vi "WPI_AnalogChannelGetOffset.vi"(8 "error in (no error)":errorcluster, 11 "AIDeviceRef":T1={"DevStatus"={"status"=FALSE, "code"=0, "source"=""}, "Analog Channel"=enum."Invalid"}) -> (0 "error out":errorcluster, 2 "Offset":dbl, 3 "AIDeviceRef":T1={"DevStatus"={"status"=FALSE, "code"=0, "source"=""}, "Analog Channel"=enum."Invalid"})   [LabVIEW 2017]
doc: "Returns the factory offset value that the A/D converter uses to scale the signal.\n\nThis software is licensed. Open the labview\\readme\\WPI Robotics Library Open Source License.txt file for more information."
uses:
  <vilib>/Rock Robotics/WPI/AnalogChannel/WPI_AnalogChannelDevRef.ctl
  <vilib>/Rock Robotics/SystemInterfaces/AI/FPGA_AIChannel.ctl
  <vilib>/Rock Robotics/SystemInterfaces/System/FPGA_SystemGet.vi
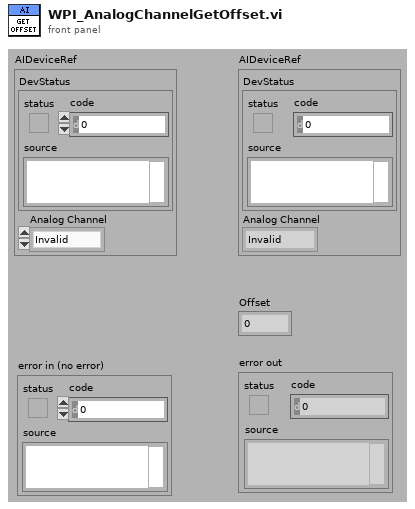
[diagram p1: front panel]
types:
  T1 = typedef "WPI_AnalogChannelDevRef.ctl" = cluster{"DevStatus":errorcluster, "Analog Channel":T2}
  T2 = typedef "FPGA_AIChannel.ctl" = enum8{"AI 0", "AI 1", "AI 2", "AI 3", "AI MXP 0", "AI MXP 1", "AI MXP 2", "AI MXP 3", "Invalid"}
  T3 = typedef "FPGA_AIDevRef.ctl" = cluster{"DevStatus":errorcluster}
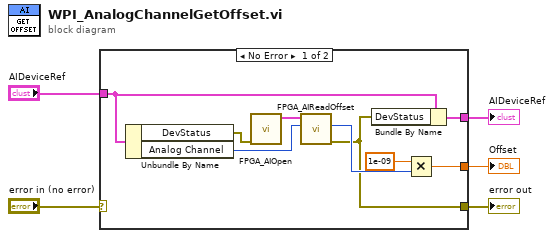
[diagram p0: block diagram]
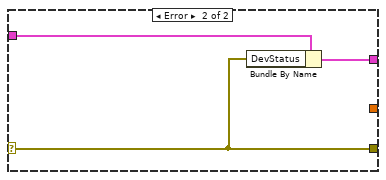
[diagram p2: hidden frame]
diagram:
  n1 = case shown="No Error" "error in (no error)" {
    selector: "error in (no error)" -> [_ w15]
    tunnel: [w7 _] -> w5
    tunnel: [w11 w17] -> w4
    tunnel: "AIDeviceRef" -> [w10 w16]
    tunnel: [w8 w15] -> w1
    frame No Error {
      n2 = Unbundle By Name(w10) -> ("DevStatus"=w14:errorcluster, "Analog Channel"=w9:T2)
      n3 = call <vilib>:"FPGA_AIOpen.vi"("error in (no error)"=w14) -> ("AI Reference out"=w13:T3)  [unwired: 2 in, 8 out]
      n4 = call <vilib>:"FPGA_AIReadOffset.vi"("Channel"=w9, "AI Reference"=w13) -> ("error out"=w8:errorcluster, "Offset"=w12:i32)  [unwired: 1 in, 7 out]
      n5 = Bundle By Name(cluster=w10, "DevStatus"=w8) -> (w11:T1)
      n6 = Multiply(x=1e-09, y=w12) -> (x*y=w7:dbl)
    }
    frame Error {
      n7 = Bundle By Name(cluster=w16, "DevStatus"=w15) -> (w17:T1)
    }
  }
  "AIDeviceRef" <- w4
  "Offset" <- w5
  "error out" <- w1
